vi "Angular Speed Ex.vi"(7 "reset? (True)":bool=TRUE, 8 "error in (no error)":errorcluster, 9 "avg on n pulses (1:no average)":i32=1, 10 "pulse/revolution (1)":dbl=1.0 format="%.2f", 11 "pulse positions [s]":dbl[](array[numeric]) format="%.2f") -> (0 "error out":errorcluster, 3 "speed profile":T1 {"speed [RPM]" format="%.2f"; "time [s]" format="%.2f"})   [LabVIEW 2017, in "SoundVib_TachProcess.lvlib"]
doc: "Computes the angular speed at each pulse edge contained in <B>pulse positions [s]</B>."
uses:
  <vilib>/addons/Sound and Vibration/Order Analysis/Tach Process/SoundVib_TachProcess.lvlib
  <vilib>/addons/Sound and Vibration/Order Analysis/Tach Process/SubVIs/speed profile.ctl
panel:
  # "Angular Speed (at edges)"
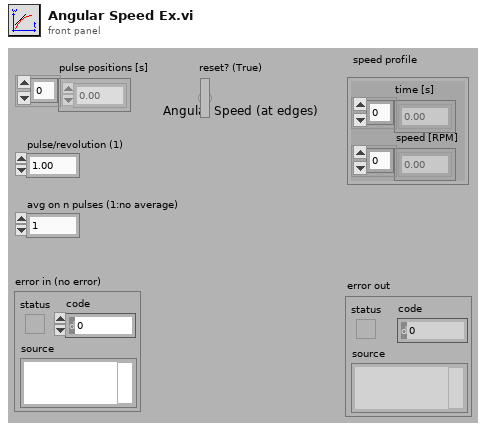
[diagram p1: front panel]
types:
  T1 = typedef "SoundVib_TachProcess.lvlib/speed profile.ctl" = cluster{"time [s]":dbl[], "speed [RPM]":dbl[]}
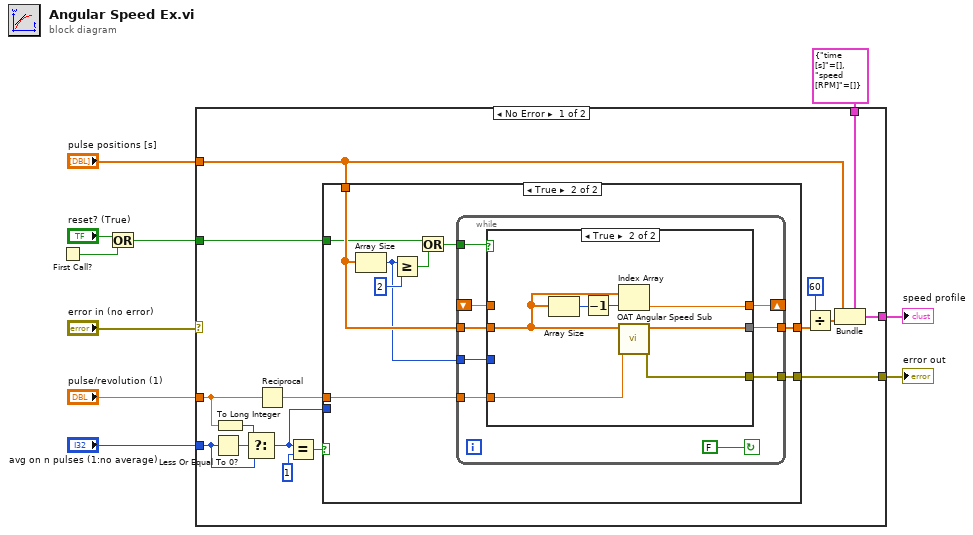
[diagram p0: block diagram]
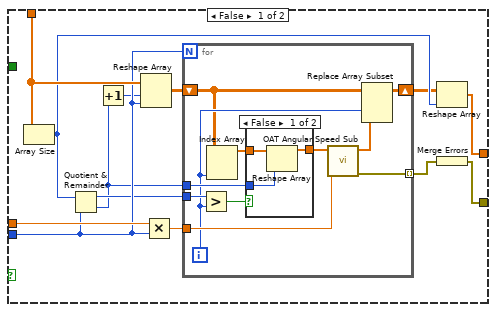
[diagram p2: hidden frame]
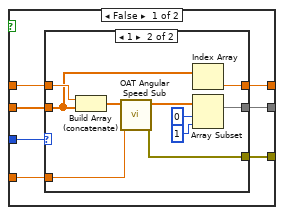
[diagram p4: hidden frame]
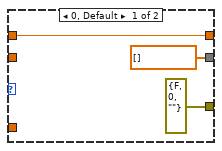
[diagram p5: hidden frame]
diagram:
  n1 = First Call?() -> (First Call?: T/F=w3:bool)
  n2 = Or(x="reset? (True)", y=w3) -> (x .or. y?=w1:bool)
  n3 = case shown="No Error" "error in (no error)" {
    selector: "error in (no error)" -> [_ w100]
    tunnel: "avg on n pulses (1:no average)" -> [w25 _]
    tunnel: "pulse positions [s]" -> [w18 _]
    tunnel: [w17 w101] -> w8
    tunnel: "pulse/revolution (1)" -> [w14 _]
    tunnel: [w13 w100] -> w6
    tunnel: T1 {"time [s]"=[], "speed [RPM]"=[]} ("speed profile") -> [w12 w101]
    tunnel: w1 -> [w11 _]
    frame No Error {
      n4 = Less Or Equal To 0?(x=w25) -> (x <= 0?=w26:bool)
      n5 = To Long Integer(number=w14) -> (32bit integer=w19:i32)
      n6 = Select(t=w19, s=w26, f=w25) -> (s? t:f=w21:i32)
      n7 = Reciprocal(x=w14) -> (1/x=w22:dbl)
      n8 = Equal?(x=w21, y=1) -> (x = y?=w23:bool)
      n9 = case shown="True" w23 {
        tunnel: w18 -> [w39 w60]
        tunnel: w22 -> [w38 w63]
        tunnel: [w29 w62] -> w15
        tunnel: w21 -> [w37 _]
        tunnel: [w27 w61] -> w13
        tunnel: w11 -> [_ w57]
        frame False {
          n10 = Array Size(array=w39) -> (size(s)=w35:i32)
          n11 = Quotient & Remainder(x=w35, y=w37) -> (x-y*floor(x/y)=w34:i32, floor(x/y)=w32:i32)
          n12 = Increment(x=w32) -> (x+1=w33:i32)
          n13 = Reshape Array(w39, w33, w37) -> (w31:dbl[][])
          n14 = Multiply(x=w38, y=w37) -> (x*y=w36:dbl)
          n15 = for {
            N: w37 -> [_]
            tunnel: w36 -> [w49]
            tunnel: w34 -> [w47]
            tunnel: w32 -> [w45]
            shift-right: [w41] -> w30
            shift-left: w31 -> [w42]
            tunnel: [w40] -> w28 mode=indexing
            i -> [w44]
            n16 = Greater?(x=w47, y=w44) -> (0:w46:bool)
            n17 = Index Array(array=w42, index (col)=w44) -> (element=w50:dbl[])  [unwired: 1 in]
            n18 = case shown="False" w46 {
              tunnel: w50 -> [w53 w54]
              tunnel: [w52 w54] -> w48
              tunnel: w45 -> [w51 _]
              frame False {
                n19 = Reshape Array(w53, w51) -> (w52:dbl[])
              }
              frame True {
              }
            }
            n20 = call <vilib>:"OAT Angular Speed Sub.vi"("deltaX"=w49, "Y[n]"=w48) -> ("error out"=w40:errorcluster, "dY/dX[n]"=w43:dbl[])  [unwired: 8 in]
            n21 = Replace Array Subset(array=w42, new element=w43, index (col)=w44) -> (w41:dbl[][])  [unwired: 1 in]
          }
          n22 = Reshape Array(w30, w35) -> (w29:dbl[])
          n23 = Merge Errors(w28) -> (w27:errorcluster)
        }
        frame True {
          n24 = Array Size(array=w60) -> (size(s)=w55:i32)
          n25 = Greater Or Equal?(x=w55, y=2) -> (x >= y?=w58:bool)
          n26 = Or(x=w57, y=w58) -> (x .or. y?=w56:bool)
          n27 = while {
            tunnel: w60 -> [w72]
            tunnel: w63 -> [w71]
            tunnel: [w70] -> w62
            tunnel: [w69] -> w61
            shift-right: [w67] -> _
            shift-left: _ -> [w66]
            tunnel: w56 -> [w65]
            tunnel: w55 -> [w64]
            stop <- FALSE continue-if-true
            n28 = case shown="True" w65 {
              tunnel: w72 -> [w77 w93]
              tunnel: w71 -> [w79 w99]
              tunnel: [w75 w97] -> w70
              tunnel: [w78 w98] -> w69
              tunnel: [w73 w94] -> w67
              tunnel: w66 -> [w76 _]
              tunnel: w64 -> [w74 _]
              frame False {
                n29 = case shown="1" w74 {
                  tunnel: w79 -> [_ w92]
                  tunnel: [errorcluster {"status"=FALSE, "code"=0, "source"=""} ("error out") w91] -> w78
                  tunnel: w77 -> [_ w83]
                  tunnel: w76 -> [w82 w90]
                  tunnel: [dbl[] [] w86] -> w75
                  tunnel: [w82 w84] -> w73
                  frame 0, Default {
                  }
                  frame 1 {
                    n30 = Build Array (concatenate)(w90, w83) -> (w85:dbl[])
                    n31 = call <vilib>:"OAT Angular Speed Sub.vi"("deltaX"=w92, "Y[n]"=w85) -> ("error out"=w91:errorcluster, "dY/dX[n]"=w89:dbl[])  [unwired: 8 in]
                    n32 = Index Array(array=w83) -> (element=w84:dbl)  [unwired: 1 in]
                    n33 = Array Subset(array=w89, index=0, length=1) -> (w86:dbl[])
                  }
                }
              }
              frame True {
                n34 = Array Size(array=w93) -> (size(s)=w96:i32)
                n35 = Decrement(x=w96) -> (x-1=w95:i32)
                n36 = Index Array(array=w93, index=w95) -> (element=w94:dbl)
                n37 = call <vilib>:"OAT Angular Speed Sub.vi"("deltaX"=w99, "Y[n]"=w93) -> ("error out"=w98:errorcluster, "dY/dX[n]"=w97:dbl[])  [unwired: 8 in]
              }
            }
          }
        }
      }
      n38 = Divide(x=60, y=w15) -> (x/y=w16:dbl[])
      n39 = Bundle(cluster=w12, "time [s]"=w18, "speed [RPM]"=w16) -> (w17:T1)
    }
    frame Error {
    }
  }
  "speed profile" <- w8
  "error out" <- w6
